vi "Custom Sorted Particle Report.vi"(6 "Min Area Size %":dbl, 8 "Max Area Size %":dbl, 9 "Particle Count Limit":dbl=inf, 10 "Pixel Measurements":T1[](array[typedef])=[35, 4, 5, 6, 7] items=["Center of Mass X", "Center of Mass Y", "First Pixel X", "First Pixel Y", "Bounding Rect Left", "Bounding Rect Top", "Bounding Rect Right", "Bounding Rect Bottom", "Max Feret Diameter Start X", "Max Feret Diameter Start Y", "Max Feret Diameter End X", "Max Feret Diameter End Y", "Max Horiz. Segment Length Left", "Max Horiz. Segment Length Right", "Max Horiz. Segment Length Row", "-", "Bounding Rect Width", "Bounding Rect Height", "Bounding Rect Diagonal", "Perimeter", "Convex Hull Perimeter", "Holes' Perimeter", "Max Feret Diameter", "Equivalent Ellipse Major Axis", "Equivalent Ellipse Minor Axis", "Equivalent Ellipse Minor Axis (Feret)", "Equivalent Rect Long Side", "Equivalent Rect Short Side", "Equivalent Rect Diagonal", "Equivalent Rect Short Side (Feret)", "Average Horiz. Segment Length", "Average Vert. Segment Length", "Hydraulic Radius", "Waddel Disk Diameter", "-", "Area", "Holes' Area", "Particle & Holes' Area", "Convex Hull Area", "Image Area", "-", "Number of Holes", "Number of Horiz. Segments", "Number of Vert. Segments", "-", "Orientation", "Max Feret Diameter Orientation", "-", "% Area/Image Area", "% Area/(Particle & Holes' Area)", "Ratio of Equivalent Ellipse Axes", "Ratio of Equivalent Rect Sides", "-", "Elongation Factor", "Compactness Factor", "Heywood Circularity Factor", "Type Factor", "-", "Sum X", "Sum Y", "Sum XX", "Sum XY", "Sum YY", "Sum XXX", "Sum XXY", "Sum XYY", "Sum YYY", "-", "Moment of Inertia XX", "Moment of Inertia XY", "Moment of Inertia YY", "Moment of Inertia XXX", "Moment of Inertia XXY", "Moment of Inertia XYY", "Moment of Inertia YYY", "Norm. Moment of Inertia XX", "Norm. Moment of Inertia XY", "Norm. Moment of Inertia YY", "Norm. Moment of Inertia XXX", "Norm. Moment of Inertia XXY", "Norm. Moment of Inertia XYY", "Norm. Moment of Inertia YYY", "Hu Moment 1", "Hu Moment 2", "Hu Moment 3", "Hu Moment 4", "Hu Moment 5", "Hu Moment 6", "Hu Moment 7"], 11 "Image in":T2) -> (2 "Particles":i32, 3 "Sorted Data":dbl[][](array[numeric]))   [LabVIEW 2015]
uses:
  <vilib>/vision/Image Controls.llb/IMAQ Image.ctl
  <vilib>/vision/NI_Vision_Development_Module.lvlib
panel:
  out "Particle Measurements (Real-World)":dbl[][](array[numeric]) format="%.2f"
  out "reversed array":cluster{"Numeric":dbl, i32}[](array[cluster])
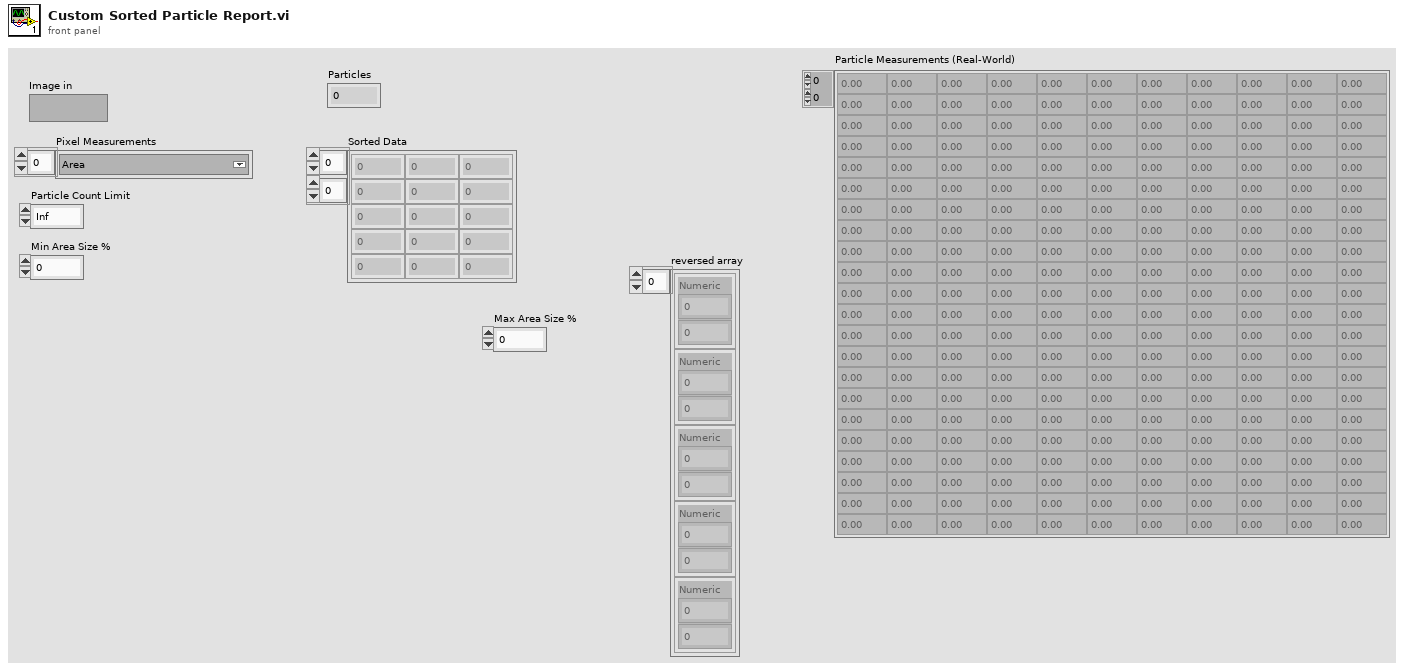
[diagram p1: front panel]
types:
  T1 = typedef "Particle Parameters" = i32
  T2 = typedef "IMAQ Image.ctl" = refnum<image>
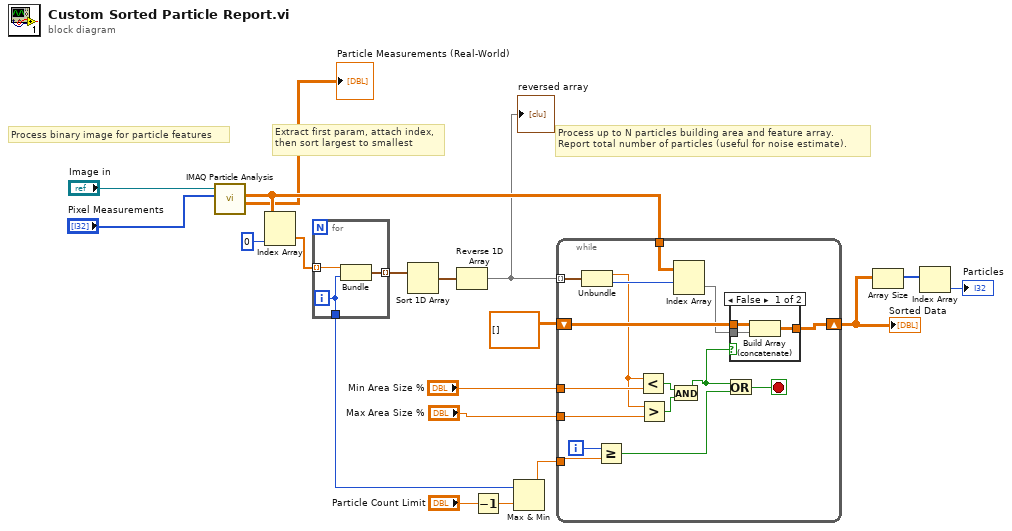
[diagram p0: block diagram]
diagram:
  # "Process up to N particles building area and feature array.\nReport total number of particles (useful for noise estimate)."
  # "Process binary image for particle features"
  # "Extract first param, attach index,\nthen sort largest to smallest"
  n1 = call "IMAQ Particle Analysis"("Pixel Measurements"="Pixel Measurements", "Image"="Image in") -> ("Particle Measurements (Real-World)"=→"Particle Measurements (Real-World)":dbl[][], "Particle Measurements (Pixels)"=w13:dbl[][])  [unwired: 3 in, 5 out]
  n2 = Index Array(array=w13, index (col)=0 ("disabled index (col)")) -> (element=w16:dbl[])  [unwired: 1 in]
  n3 = for {
    tunnel: w16 -> [w22] mode=indexing
    tunnel: [w21] -> w17 mode=indexing
    tunnel: [w20] -> w3
    i -> [w20]
    n4 = Bundle("Numeric"=w22, w20) -> (w21:cluster{"Numeric":dbl, i32})  [unwired: 1 out]
  }
  n5 = Sort 1D Array(array=w17) -> (sorted array=w18:cluster{"Numeric":dbl, i32}[])
  n6 = Reverse 1D Array(array=w18) -> (reversed array=w6:cluster{"Numeric":dbl, i32}[])
  "reversed array" <- w6
  n7 = Decrement(x="Particle Count Limit") -> (x-1=w4:dbl)
  n8 = Max & Min(x=w3, y=w4) -> (min(x,y)=w5:dbl)  [unwired: 1 out]
  n9 = while {
    tunnel: w13 -> [w37]
    tunnel: w6 -> [w36] mode=indexing
    shift-right: [w33] -> w9
    shift-left: dbl[][] [] -> [w35]
    tunnel: w5 -> [w31]
    tunnel: "Min Area Size %" -> [w30]
    tunnel: "Max Area Size %" -> [w26]
    i -> [w32]
    stop <- w28 stop-if-true
    n10 = Unbundle(w36) -> ("Numeric"=w27:dbl, w38:i32)
    n11 = Greater Or Equal?(x=w32, y=w31) -> (x >= y?=w29:bool)
    n12 = Less?(x=w27, y=w30) -> (x < y?=w25:bool)
    n13 = Greater?(x=w27, y=w26) -> (0:w24:bool)
    n14 = And(x=w25, y=w24) -> (x .and. y?=w23:bool)
    n15 = Index Array(array=w37, index (row)=w38) -> (element=w34:dbl[])  [unwired: 1 in]
    n16 = Or(x=w23, y=w29) -> (x .or. y?=w28:bool)
    n17 = case shown="False" w23 {
      tunnel: w35 -> [w41 w42]
      tunnel: w34 -> [w40 _]
      tunnel: [w39 w42] -> w33
      frame False {
        n18 = Build Array (concatenate)(w41, w40) -> (w39:dbl[][])
      }
      frame True {
      }
    }
  }
  "Sorted Data" <- w9
  n19 = Array Size(array=w9) -> (size(s)=w8:i32[])
  n20 = Index Array(array=w8) -> (element=→"Particles":i32)  [unwired: 1 in]
